vi "Find Stack Start Index.vi"(8 "error in (no error)":errorcluster, 11 "Image Array":T1[](array[typedef])) -> (0 "error out":errorcluster, 3 "Start Index":i32)   [LabVIEW 2013]
uses:
  <vilib>/vision/Image Controls.llb/IMAQ Image.ctl
  <vilib>/vision/NI_Vision_Development_Module.lvlib
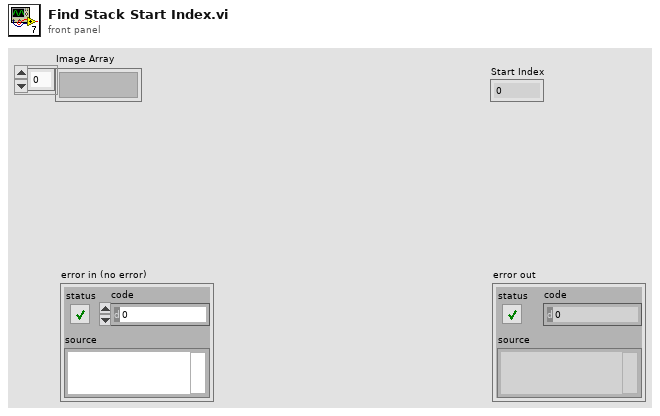
[diagram p1: front panel]
types:
  T1 = typedef "IMAQ Image.ctl" = refnum<image>
  T2 = cluster{"Position":cluster{"X":sgl, "Y":sgl}, "Orientation":dbl, "Major Radius":dbl, "Minor Radius":dbl, "Score":dbl}[]
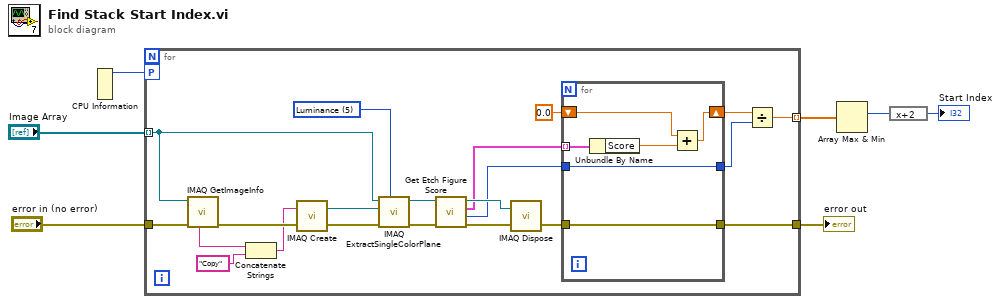
[diagram p0: block diagram]
diagram:
  n1 = CPU Information() -> (4:w3:i32)  [unwired: 3 out]
  n2 = for {
    tunnel: "Image Array" -> [w10] mode=indexing
    tunnel: "error in (no error)" -> [w28]
    tunnel: [w15] -> w5
    tunnel: [w14] -> w4 mode=indexing
    workers-P: w3 -> [_]
    w8 = 5 items=["Red", "Green", "Blue", "Hue", "Saturation", "Luminance", "Value", "Intensity"] ("Color Plane")
    n3 = call "IMAQ GetImageInfo"("error in (no error)"=w28, "Image"=w10) -> ("error out"=w25:errorcluster, "Image Name"=w27:string)  [unwired: 2 in, 6 out]
    n4 = Concatenate Strings(w27, "Copy" ("string")) -> (w24:string)
    n5 = call "IMAQ Create"("Image Name"=w24, "error in (no error)"=w25) -> ("New Image"=w9:T1, "error out"=w13:errorcluster)  [unwired: 3 in]
    n6 = call "IMAQ ExtractSingleColorPlane"("Color Plane"=w8, "error in (no error)"=w13, "Image Dst"=w9, "Image Src"=w10) -> ("error out"=w12:errorcluster, "Image Dst Out"=w11:T1)  [unwired: 6 in]
    n7 = call "Get Etch Figure Score.vi"("error in"=w12, "Image In"=w11) -> ("error out"=w23:errorcluster, "Number of Matches"=w17:i32, "Ellipses"=w21:T2, "Image Out"=w22:T1)  [unwired: 6 in]
    n8 = call "IMAQ Dispose"("Image"=w22, "error in (no error)"=w23) -> ("error out"=w20:errorcluster)  [unwired: 4 in]
    n9 = for {
      tunnel: w21 -> [w34] mode=indexing
      tunnel: w20 -> [w33]
      tunnel: [w33] -> w15
      shift-right: [w31] -> w18
      shift-left: 0.0 -> [w30]
      tunnel: w17 -> [w29]
      tunnel: [w29] -> w16
      n10 = Unbundle By Name(w34) -> ("Score"=w32:dbl)
      n11 = Add(x=w30, y=w32) -> (x+y=w31:dbl)
    }
    n12 = Divide(x=w18, y=w16) -> (x/y=w14:dbl)
  }
  "error out" <- w5
  n13 = Array Max & Min(array=w4) -> (max index (indices)=w1:i32)  [unwired: 3 out]
  n14 = expression code="x+2"(w1) -> (→"Start Index":i32)
